vi "Get Path.vi"(8 "error in (no error)":errorcluster, 11 "SequenceFile in":refnum<class "SequenceFile.lvclass">) -> (0 "error out":errorcluster, 2 "Path":path, 3 "SequenceFile out":refnum<class "SequenceFile.lvclass">)   [LabVIEW 2020, in "TSnax.lvlib" / "SequenceFile.lvclass"]
uses:
  SequenceFile.lvclass
  SequenceFile.lvclass/SequenceFile.ctl
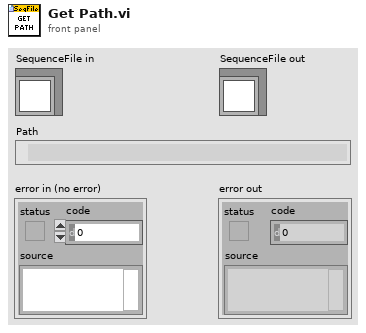
[diagram p1: front panel]
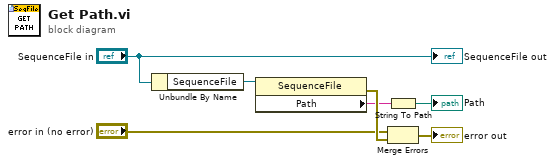
[diagram p0: block diagram]
diagram:
  n1 = Unbundle By Name("SequenceFile in") -> ("SequenceFile"=w4:refnum<k7>)
  n2 = property class="SequenceFile"(reference=w4) -> (error out=w7:errorcluster, "Path"=w3:string)  [unwired: 1 in, 1 out]
  n3 = String To Path(string=w3) -> (path=→"Path":path)
  n4 = Merge Errors("error in (no error)", w7) -> (→"error out":errorcluster)
  "SequenceFile out" <- "SequenceFile in"
